vi "gen_drive_waveform.vi"(9 "TxRxParams":T1={"sample rate"=1000000.0, "Transmit frequency"=25000.0, "Transmit amplitude"=1.577, "sample rate digital out"=40000.0, "TX cycles"=600, "sample rate DAQ1"=1000000.0, "Receive frequency"=75000.0, "Receive range"=1.0, "TX harmonics"=[50000.0, 75000.0, 100000.0, 125000.0, 150000.0, 175000.0, 200000.0, 225000.0]} {"TX harmonics" format="%#_6p"; "Receive frequency" format="%#_6p"; "sample rate DAQ1" format="%#_6p"; "sample rate digital out" format="%#_6p"; "Transmit frequency" format="%#_6p"; "sample rate" format="%#_6p"}, 11 "no of cycles":dbl=6000.0) -> (0 "signal out":waveform(dbl))   [LabVIEW 2021]
uses:
  <vilib>/measure/NI_MABase.lvlib
panel:
  out "sample rate (from global)":dbl=500000.0 format="%#_6p"
  out "Transmit amplitude (from global)":dbl=3.3
  out "Transmit frequency (from global)":dbl=25000.0 format="%#_6p"
  out "Sample points per cycle":dbl
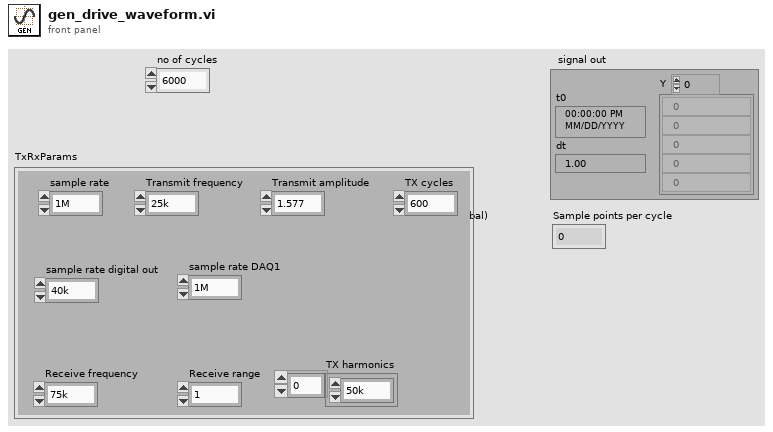
[diagram p1: front panel]
types:
  T1 = cluster{"sample rate":dbl, "Transmit frequency":dbl, "Transmit amplitude":dbl, "sample rate digital out":dbl, "TX cycles":i32, "sample rate DAQ1":dbl, "Receive frequency":dbl, "Receive range":dbl, "TX harmonics":dbl[]}
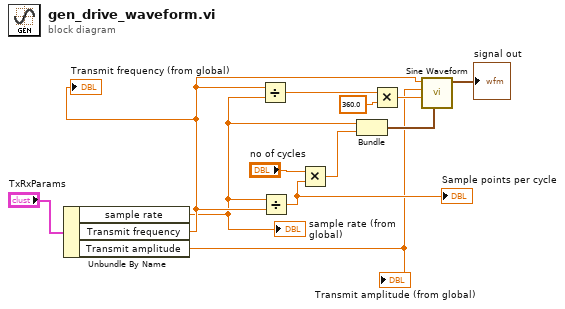
[diagram p0: block diagram]
diagram:
  n1 = Unbundle By Name("TxRxParams") -> ("sample rate"=w1:dbl, "Transmit frequency"=w3:dbl, "Transmit amplitude"=w2:dbl)
  "Transmit frequency (from global)" <- w3
  "Transmit amplitude (from global)" <- w2
  "sample rate (from global)" <- w1
  n2 = Divide(x=w3, y=w1) -> (x/y=w11:dbl)
  n3 = Divide(x=w1, y=w3) -> (x/y=w6:dbl)
  "Sample points per cycle" <- w6
  n4 = Multiply(x="no of cycles", y=w6) -> (x*y=w5:dbl)
  n5 = Bundle("sample rate"=w1, w5) -> (w12:cluster{"sample rate":dbl, dbl})  [unwired: 1 in]
  n6 = Multiply(x=w11, y=360.0) -> (x*y=w9:dbl)
  n7 = call <vilib>:"Sine Waveform.vi"("sampling info"=w12, "phase"=w9, "amplitude"=w2, "frequency"=w3) -> ("signal out"=→"signal out":waveform(dbl))  [unwired: 6 in, 1 out]
